vi "LoggingData.vi"(8 "error in (no error)":errorcluster, 10 "Start time":u32, 11 "Byte Stream File in":refnum<file>) -> (0 "error out":errorcluster, 3 "Byte Stream File out":refnum<file>)   [LabVIEW 2017]
uses:
  <vilib>/Rock Robotics/WPI/DriverStation/WPI_DriverStationRobotMode2.ctl
  Framework/Robot Global Data.vi
  Drive/Implementation/Drive Published Globals.vi
  <vilib>/NI_Real-Time Target Support.lvlib
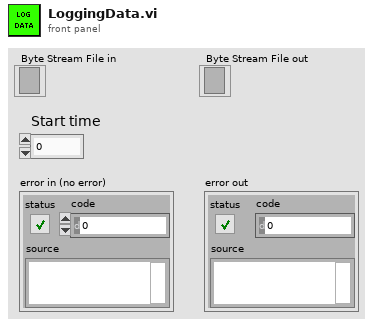
[diagram p1: front panel]
types:
  T1 = typedef "WPI_DriverStationRobotMode2.ctl" = enum16{"Autonomous Disabled", "Autonomous Enabled", "Teleop Disabled", "Teleop Enabled", "Disconnected", "Finish", "Test Disabled", "Test Enabled", "Emergency Stopped"}
  T2 = typedef "Z900_navX_Flags_OpStatusTypeDef.ctl" = u8
  T3 = typedef "Z900_navX_Flags_CalibrationStatusTypeDef.ctl" = u8
  T4 = cluster{"Update Rate Hz":u8, "Accelerometer Full-Scale Range":u8, "Gyro Full-Scale Range":u16, "OP Status":T2, "Calibration Status":T3, "Sensor Status":cluster{"MOVING":bool, "YAW_STABLE":bool, "MAG_DISTURBANCE":bool, "ALTITUDE_VALID":bool, "SEALEVEL_PRESS_SET":bool, "FUSED_HEADING_VALID":bool}, "Self Test Status":cluster{"Gyro Passed":bool, "Accel Passed":bool, "Mag Passed":bool, "Baro Passed":bool, "Complete":bool}}
  T5 = cluster{"MOVING":bool, "YAW_STABLE":bool, "MAG_DISTURBANCE":bool, "ALTITUDE_VALID":bool, "SEALEVEL_PRESS_SET":bool, "FUSED_HEADING_VALID":bool}
  T6 = cluster{"Yaw":dbl, "Roll":dbl, "Pitch":dbl, "Heading":dbl, "Fused Heading":dbl}
  T7 = typedef "NI_Real-Time Target Support.lvlib/RT CPU Load.ctl" = cluster{"Total (%)":dbl, "Time Critical (%)":dbl, "Timed Structures (%)":dbl, "High (%)":dbl, "Above Normal (%)":dbl, "Normal (%)":dbl, "Background (%)":dbl, "Idle (%)":dbl, "ISR (%)":dbl}
  T8 = cluster{"LinearAcceleration X":dbl, "LinearAcceleration Y":dbl, "LinearAcceleration Z":dbl}
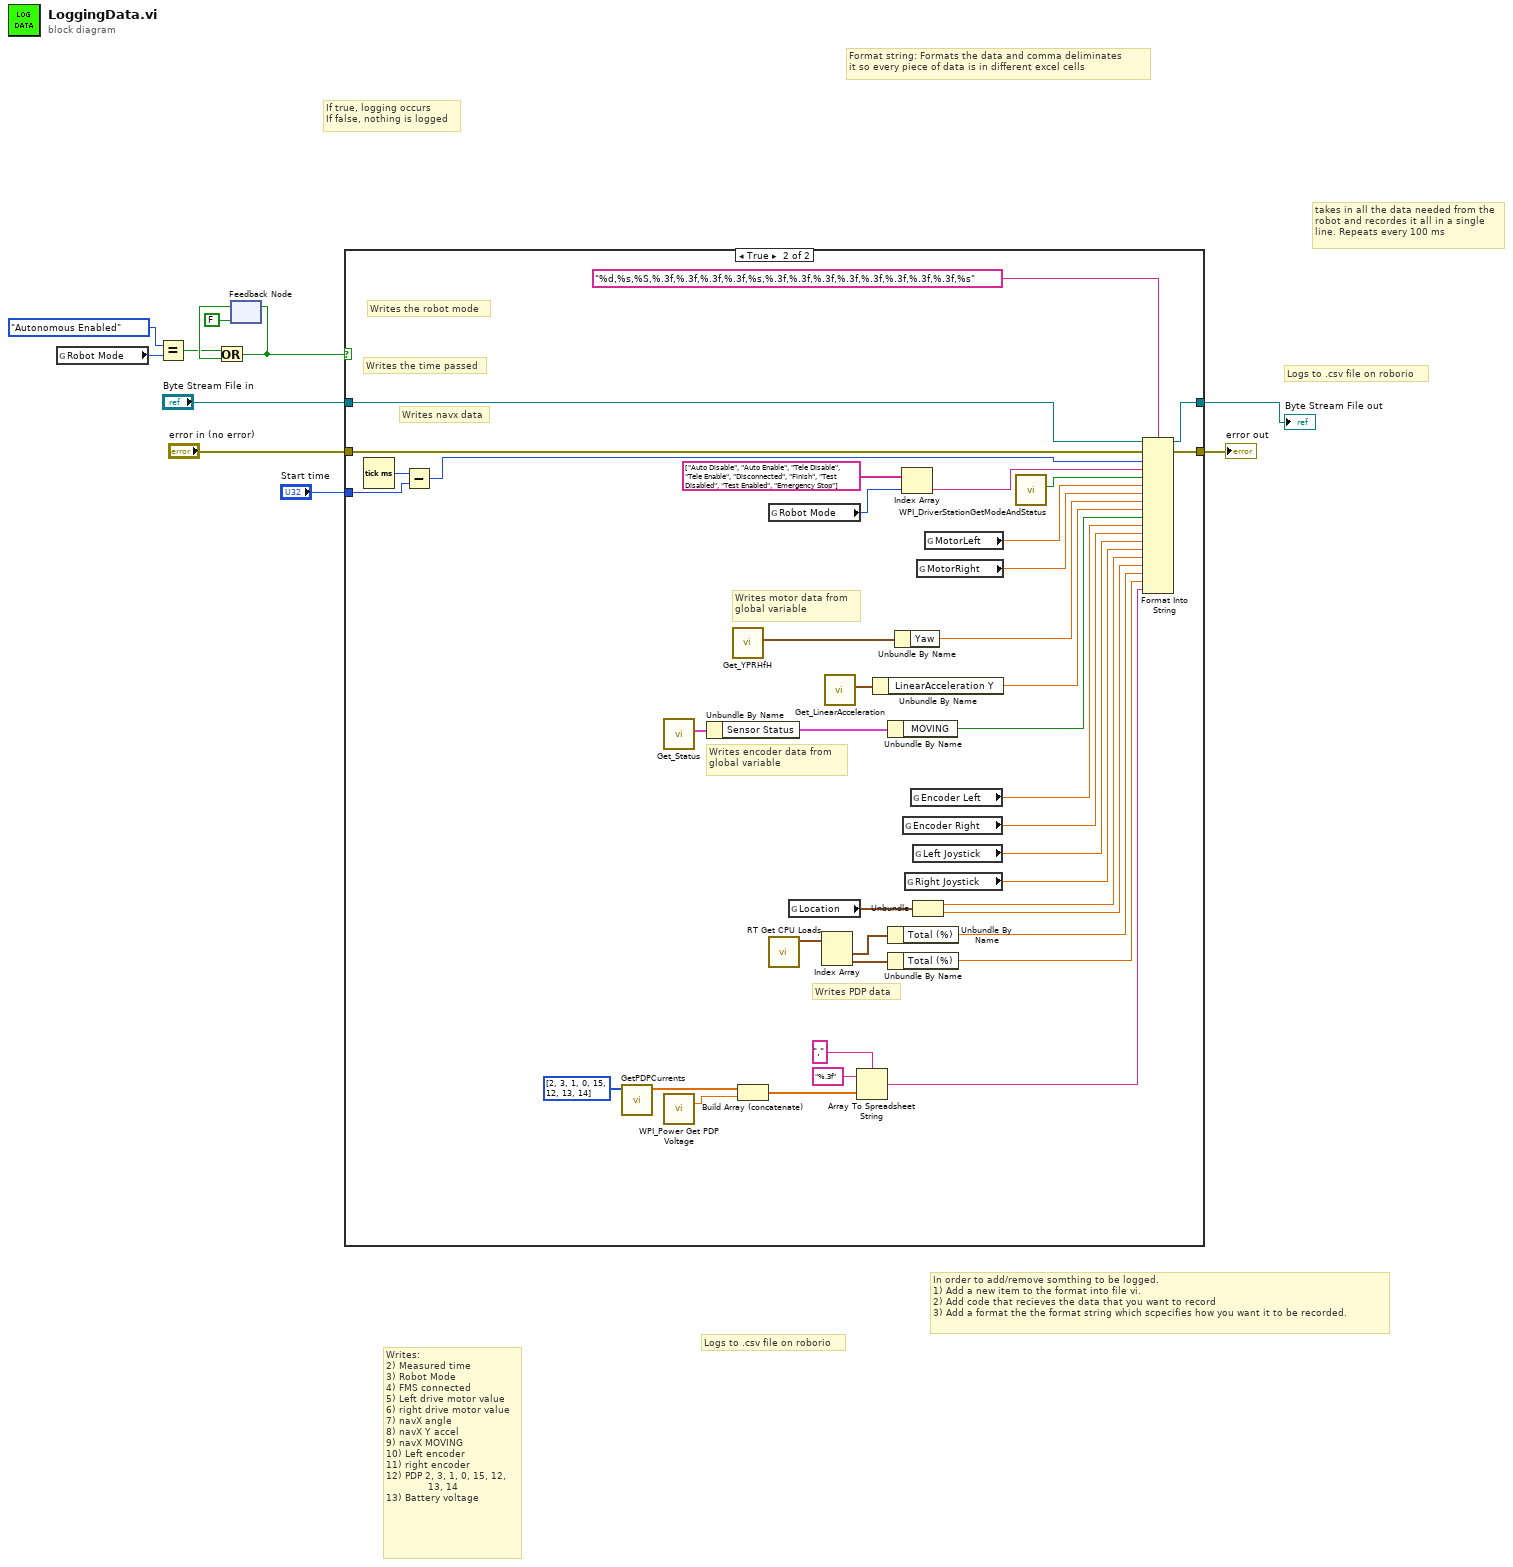
[diagram p0: block diagram]
diagram:
  # "Format string: Formats the data and comma deliminates \nit so every piece of data is in different excel cells"
  # "In order to add/remove somthing to be logged.\n1) Add a new item to the format into file vi.\n2) Add code that recieves the data that you want to record\n3) Add a format the the format string which scpecifies how you want it to be recorded."
  # "Logs to .csv file on roborio"
  # "If true, logging occurs\nIf false, nothing is logged"
  # "Writes:\n2) Measured time\n3) Robot Mode\n4) FMS connected\n5) Left drive motor value\n6) right drive motor value\n7) navX angle\n8) navX Y accel\n9) navX MOVING\n10) Left encoder\n11) right encoder\n12) PDP 2, 3, 1, 0, 15, 12,\n              13, 14\n13) Battery voltage"
  # "takes in all the data needed from the robot and recordes it all in a single line. Repeats every 100 ms"
  # "Logs to .csv file on roborio"
  n1 = global read "Robot Global Data.vi" "Robot Mode"() -> (w1:T1)
  n2 = Equal?(x=WPI_DriverStationRobotMode2."Autonomous Enabled", y=w1) -> (x = y?=w8:bool)
  n3 = feedback #1(FALSE) -> (w9:bool)
  n4 = Or(x=w8, y=w9) -> (x .or. y?=w11:bool)
  n5 = feedback-in #1(w11) -> ()
  n6 = case shown="True" w11 {
    tunnel: "error in (no error)" -> [w12 w37]
    tunnel: "Byte Stream File in" -> [w13 w39]
    tunnel: [w13 w40] -> w3
    tunnel: [w12 w38] -> w4
    tunnel: "Start time" -> [_ w53]
    frame False {
    }
    frame True {
      # "Writes the time passed"
      # "Writes the robot mode"
      # "Writes motor data from\nglobal variable"
      # "Writes navx data"
      # "Writes encoder data from \nglobal variable"
      # "Writes PDP data"
      n7 = Tick Count (ms)() -> (millisecond timer value=w49:u32)
      n8 = Subtract(x=w49, y=w53) -> (x-y=w36:u32)
      n9 = call "GetPDPCurrents.vi"("Channels"=i32[] [2, 3, 1, 0, 15, 12, 13, 14]) -> ("Currents"=w45:dbl[])  [unwired: 10 in]
      n10 = call <vilib>:"Get_Status.vi"() -> ("Status"=w41:T4)  [unwired: 11 in]
      n11 = call <vilib>:"WPI_Power Get PDP Voltage.vi"() -> ("voltage (V)"=w50:dbl)  [unwired: 14 in, 1 out]
      n12 = Unbundle By Name(w41) -> ("Sensor Status"=w51:T5)
      n13 = call <vilib>:"Get_YPRHfH.vi"() -> ("YRPHfH"=w43:T6)  [unwired: 11 in]
      n14 = Build Array (concatenate)(w45, w50) -> (w46:dbl[])
      n15 = global read "Robot Global Data.vi" "Robot Mode"() -> (w21:T1)
      n16 = call <vilib>:"RT Get CPU Loads.vi"() -> ("CPU loads"=w25:T7[])  [unwired: 10 in, 1 out]
      n17 = global read "Drive Published Globals.vi" "Location"() -> (w18:cluster{dbl, dbl})
      n18 = Index Array(array=w25) -> (element #1=w26:T7, element #2=w27:T7)  [unwired: 2 in]
      n19 = call <vilib>:"Get_LinearAcceleration.vi"() -> ("Linear Acceleration"=w42:T8)  [unwired: 11 in]
      n20 = Array To Spreadsheet String(delimiter (Tab)=",", array=w46, 3:"%.3f" ("format string")) -> (spreadsheet string=w22:string)
      n21 = Unbundle By Name(w42) -> ("LinearAcceleration Y"=w32:dbl)
      n22 = Unbundle By Name(w51) -> ("MOVING"=w31:bool)
      n23 = Unbundle By Name(w26) -> ("Total (%)"=w24:dbl)
      n24 = Unbundle By Name(w27) -> ("Total (%)"=w23:dbl)
      n25 = Unbundle By Name(w43) -> ("Yaw"=w33:dbl)
      n26 = Index Array(array=string[] ["Auto Disable", "Auto Enable", "Tele Disable", "Tele Enable", "Disconnected", "Finish", "Test Disabled", "Test Enabled", "Emergency Stop"], index=w21) -> (element=w35:string)
      n27 = global read "Drive Published Globals.vi" "Encoder Right"() -> (w16:dbl)
      n28 = global read "Robot Global Data.vi" "Right Joystick"() -> (w15:dbl)
      n29 = global read "Drive Published Globals.vi" "Encoder Left"() -> (w17:dbl)
      n30 = global read "Robot Global Data.vi" "Left Joystick"() -> (w14:dbl)
      n31 = Unbundle(w18) -> (w29:dbl, w28:dbl)
      n32 = global read "Drive Published Globals.vi" "MotorRight"() -> (w19:dbl)
      n33 = global read "Drive Published Globals.vi" "MotorLeft"() -> (w20:dbl)
      n34 = call <vilib>:"WPI_DriverStationGetModeAndStatus.vi"() -> ("FMS Attached"=w34:bool)  [unwired: 10 in, 1 out]
      n35 = Format Into String(format string="%d,%s,%S,%.3f,%.3f,%.3f,%.3f,%s,%.3f,%.3f,%.3f,%.3f,%.3f,%.3f,%.3f,%.3f,%s", initial string=w39, error in=w37, w36, w35, w34, w20, w19, w33, w32, w31, w17, w16, w14, w15, w29, w28, w24, w23, w22) -> (resulting string=w40:refnum<file>, error out=w38:errorcluster)
    }
  }
  "Byte Stream File out" <- w3
  "error out" <- w4
